vi "Destructor.vi"(8 "error in (no error)":errorcluster, 11 "Observer in":refnum<class "Observer.lvclass">) -> (0 "error out":errorcluster, 3 "Observer out":refnum<class "Observer.lvclass">)   [LabVIEW 2013, in "Observer.lvclass"]
uses:
  Observer.lvclass
  Observer.lvclass/Observer.ctl
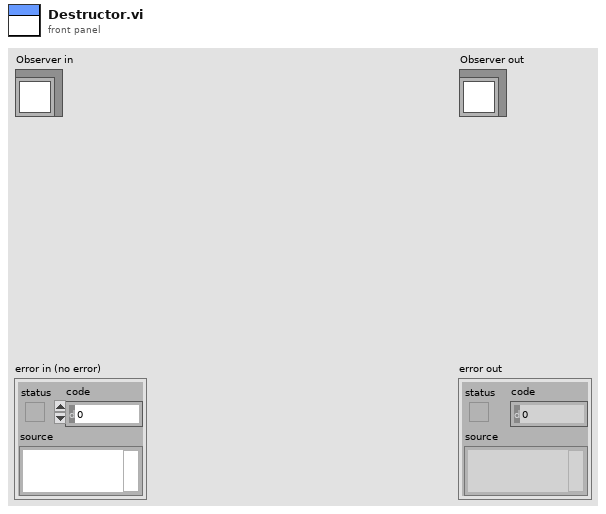
[diagram p1: front panel]
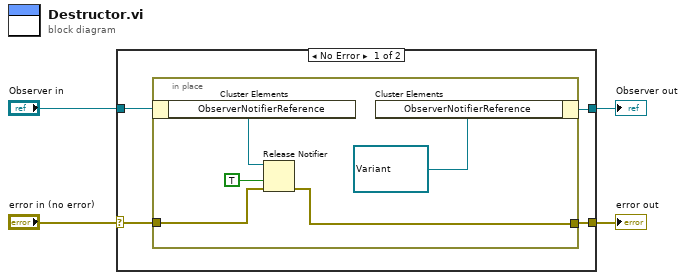
[diagram p0: block diagram]
diagram:
  n1 = case shown="No Error" "error in (no error)" {
    selector: "error in (no error)" -> [w8 w15]
    tunnel: [w7 w15] -> w1
    tunnel: [w5 w14] -> w3
    tunnel: "Observer in" -> [w6 w14]
    frame No Error {
      n2 = in-place {
        in-place-border: w8 -> [w13]
        in-place-border: [w11] -> w7
        n3 = in-place-cluster #1(w6) -> ("ObserverNotifierReference"=w12:refnum<notifier>)
        n4 = Release Notifier(notifier=w12, force destroy? (F)=TRUE, error in (no error)=w13) -> (error out=w11:errorcluster)  [unwired: 2 out]
        n5 = in-place-cluster #1("ObserverNotifierReference"=refnum<notifier> refnum ("DataNotifierReference")) -> (w5:refnum<class "Observer.lvclass">)
      }
    }
    frame Error {
    }
  }
  "error out" <- w1
  "Observer out" <- w3
